vi "Write Include Result.vi"(8 "error in (no error)":errorcluster, 10 "Include Result":bool, 11 "JsonReportPlugin in":refnum<class "JsonReportPlugin.lvclass">) -> (0 "error out":errorcluster, 3 "JsonReportPlugin out":refnum<class "JsonReportPlugin.lvclass">)   [LabVIEW 2015, in "JsonReportPlugin.lvclass"]
uses:
  JsonReportPlugin.lvclass
  JsonReportPlugin.lvclass/JsonReportPlugin.ctl
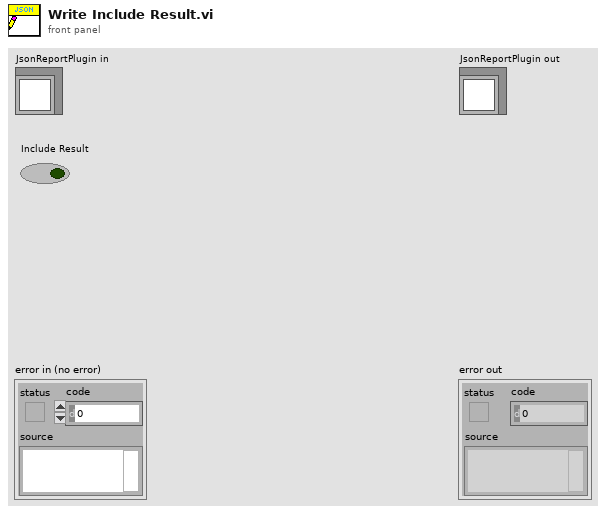
[diagram p1: front panel]
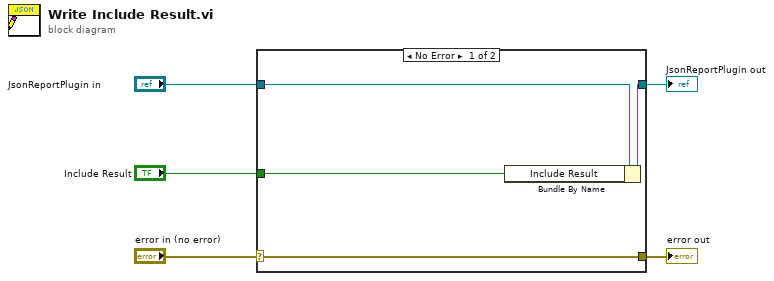
[diagram p0: block diagram]
diagram:
  n1 = case shown="No Error" "error in (no error)" {
    selector: "error in (no error)" -> [w9 w10]
    tunnel: [w9 w10] -> w4
    tunnel: [w7 w11] -> w2
    tunnel: "JsonReportPlugin in" -> [w8 w11]
    tunnel: "Include Result" -> [w6 _]
    frame No Error {
      n2 = Bundle By Name(cluster=w8, "Include Result"=w6) -> (w7:refnum<class "JsonReportPlugin.lvclass">)
    }
    frame Error {
    }
  }
  "error out" <- w4
  "JsonReportPlugin out" <- w2
